vi "onPrevious.vi"(8 "error in (no error)":errorcluster, 10 "Player In":refnum<class "Player.lvclass">, 11 "ReadyState in":refnum<class "ReadyState.lvclass">) -> (0 "error out":errorcluster, 1 "String":string, 2 "Player In 2":refnum<class "Player.lvclass">, 3 "ReadyState out":refnum<class "ReadyState.lvclass">)   [LabVIEW 2017, in "ReadyState.lvclass"]
uses:
  ReadyState.lvclass
  Player Class/Player.lvclass
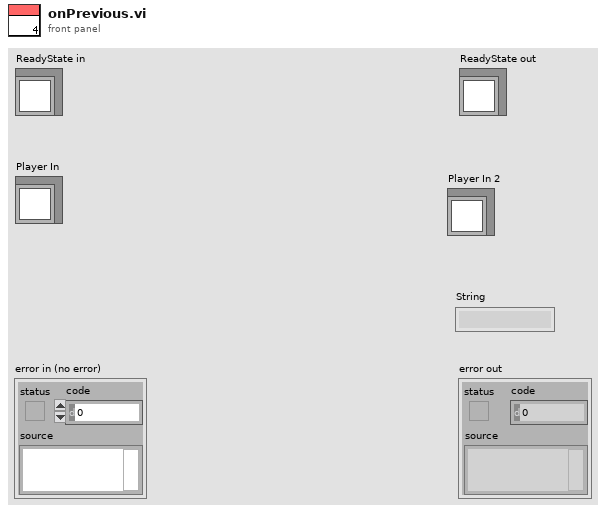
[diagram p1: front panel]
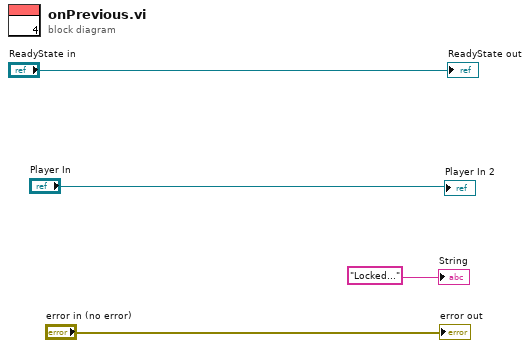
[diagram p0: block diagram]
diagram:
  "error out" <- "error in (no error)"
  "ReadyState out" <- "ReadyState in"
  "String" <- "Locked..." ("String")
  "Player In 2" <- "Player In"
